vi "Memory.Pointer.Read.1D.Bool.No Check.vi"(7 "count":u64 format="%d elements", 8 "error in (no error)":errorcluster, 9 "offset (0)":u64 format="%d bytes", 10 "buffer in":bool[](array[boolean]), 11 "pointer in":refnum<class "Memory.Pointer.lvclass">) -> (0 "error out":errorcluster, 1 "offset out":u64 format="%d bytes", 2 "buffer out":bool[](array[boolean]), 3 "pointer out":refnum<class "Memory.Pointer.lvclass">)   [LabVIEW 2016, in "Memory.lvlib" / "Memory.Pointer.lvclass"]
doc: "Reads <b>count</b> elements from the address specified by <b>pointer + offset</b> into the provided <b>buffer</b>.\n\n<b>Note:</b> This VI is <b>unsafe</b>.\n\nUnsafe means that it does not evaluate the size parameter of <b>pointer</b> to ensure that is inbounds of allocated memory before peforming a memory read/write. Reading/writing more data to a pointer than it has allocated can corrupt or crash LabVIEW. Only use this VI in scenarios where the <b>pointer</b> has been validated to be allocated to a correct size before calling this VI."
uses:
  Memory.Pointer.lvclass
  Memory.Pointer.lvclass/Memory.Pointer.ctl
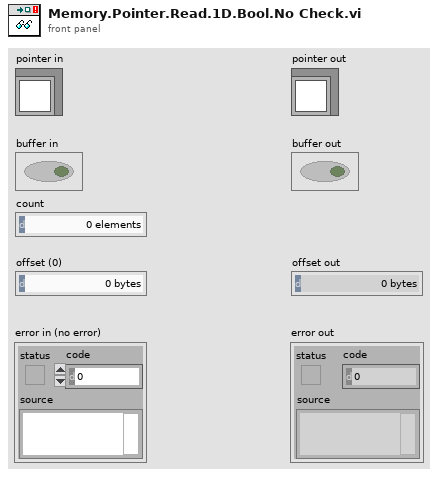
[diagram p1: front panel]
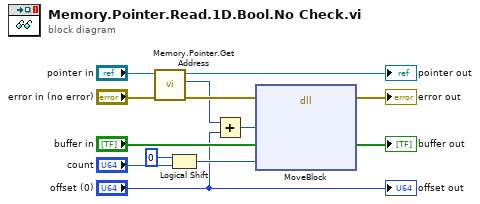
[diagram p0: block diagram]
diagram:
  n1 = call "Memory.Pointer.Get Address.vi"("Pointer in"="pointer in") -> ("address"=w1:u64, "Pointer out"=→"pointer out":refnum<class "Memory.Pointer.lvclass">)  [unwired: 9 in]
  n2 = Logical Shift(y=i16 0, x="count") -> (x << y=w6:u64)
  n3 = Add(x=w1, y="offset (0)") -> (x+y=w4:u64)
  n4 = dll-call lib="LabVIEW" fn="MoveBlock"(error in="error in (no error)", "src"=w4, "dst"="buffer in", "size"=w6) -> (error out=→"error out":errorcluster, "dst"=→"buffer out":bool[])  [unwired: 5 in, 1 out]
  "offset out" <- "offset (0)"
